vi "RichToFlatcif_manager_PluginType.vi"(5 "OutputClusterType":T1, 11 "InputCluster":T4) -> (3 "OutputCluster":T1)   [LabVIEW 2021, in "CIF_Launcher_client.lvlib"]
uses:
  CIF_Launcher_client.lvlib
  cif_manager_PluginType.ctl
  cif_common_ShortVersion.ctl
  cif_manager_PluginMetadata.ctl
  cif_manager_PluginType_Flat.ctl
  cif_common_ShortVersion_Flat.ctl
  cif_manager_PluginMetadata_Flat.ctl
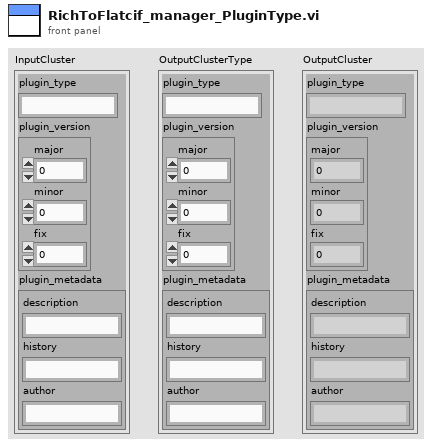
[diagram p1: front panel]
types:
  T1 = typedef "CIF_Launcher_client.lvlib/cif_manager_PluginType_Flat.ctl" = cluster{"plugin_type":string, "plugin_version":T2, "plugin_metadata":T3}
  T2 = typedef "CIF_Launcher_client.lvlib/cif_common_ShortVersion_Flat.ctl" = cluster{"major":u32, "minor":u32, "fix":u32}
  T3 = typedef "CIF_Launcher_client.lvlib/cif_manager_PluginMetadata_Flat.ctl" = cluster{"description":string, "history":string, "author":string}
  T4 = typedef "CIF_Launcher_client.lvlib/cif_manager_PluginType.ctl" = cluster{"plugin_type":string, "plugin_version":T5, "plugin_metadata":T6}
  T5 = typedef "CIF_Launcher_client.lvlib/cif_common_ShortVersion.ctl" = cluster{"major":u32, "minor":u32, "fix":u32}
  T6 = typedef "CIF_Launcher_client.lvlib/cif_manager_PluginMetadata.ctl" = cluster{"description":string, "history":string, "author":string}
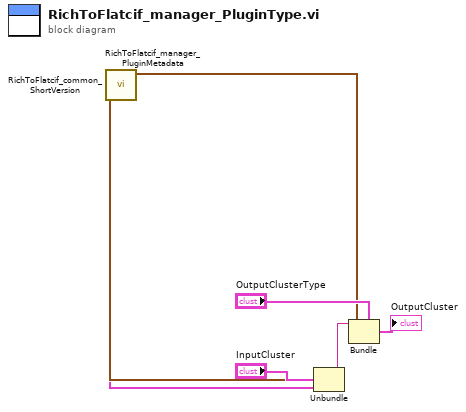
[diagram p0: block diagram]
diagram:
  n1 = Unbundle "Unbundle"("InputCluster") -> ("plugin_type"=w5:string, "plugin_version"=w4:T5, "plugin_metadata"=w2:T6)
  n2 = call "RichToFlatcif_manager_PluginMetadata.vi"("InputCluster"=w2) -> ("OutputCluster"=w1:T3)  [unwired: 10 in]
  n3 = call "RichToFlatcif_common_ShortVersion.vi"("InputCluster"=w4) -> ("OutputCluster"=w3:T2)  [unwired: 10 in]
  n4 = Bundle "Bundle"(cluster="OutputClusterType", "plugin_type"=w5, "plugin_version"=w3, "plugin_metadata"=w1) -> (→"OutputCluster":T1)
